vi "Expt_5_Transmitter_1.vi"() -> ()   [LabVIEW 2022 SP3]
uses:
  <instrlib>/niUSRP/niUSRP Write Tx Data (CDB).vi
  <vilib>/Analysis/NI_AALPro.lvlib
  <vilib>/measure/NI_MABase.lvlib
panel:
  out "Array 3":bool[](array[boolean])
  out "Digital Signal":dbl[](graph)
  out "Signal Without AWGN":dbl[](graph)
  out "XY Graph":cluster{i32[], i32[]}(graph)
  out "Array 2":i32[](array[numeric])
  out "Array":i32[](array[numeric])
  out "Numeric":dbl
  out "Signal With AWGN":waveform(dbl)[](graph)
  in  "active antenna":string
  in  "gain":dbl format="%#_6f"
  in  "carrier frequency":dbl=100000.0 format="%#_6p"
  in  "IQ rate":dbl=100000.0 format="%#_6p"
  in  "device names":refnum<k15>
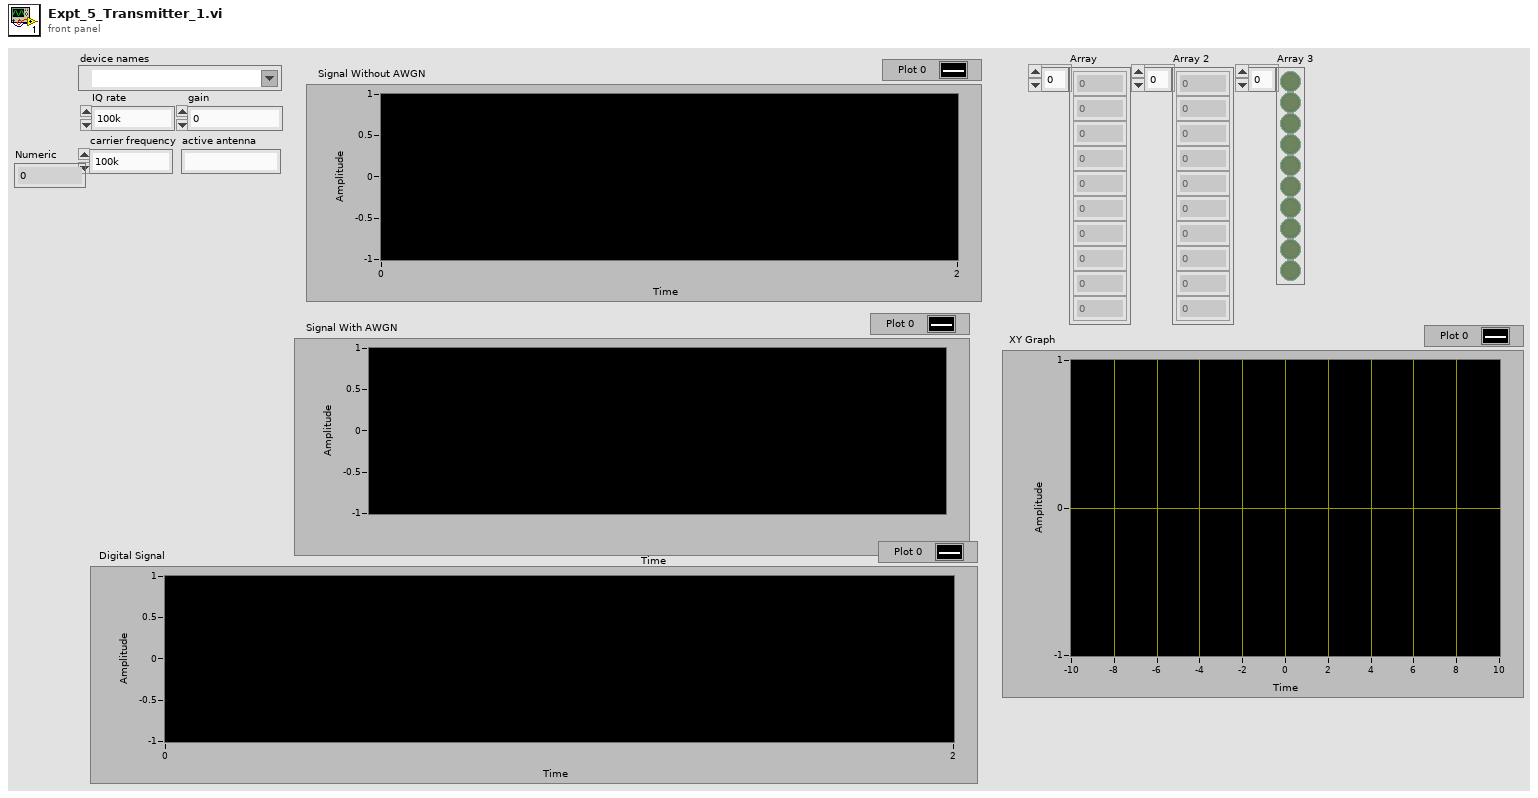
[diagram p1: front panel]
types:
  T1 = enum16{"sine", "cosine", "triangle", "square", "sawtooth", "increasing ramp", "decreasing ramp"}
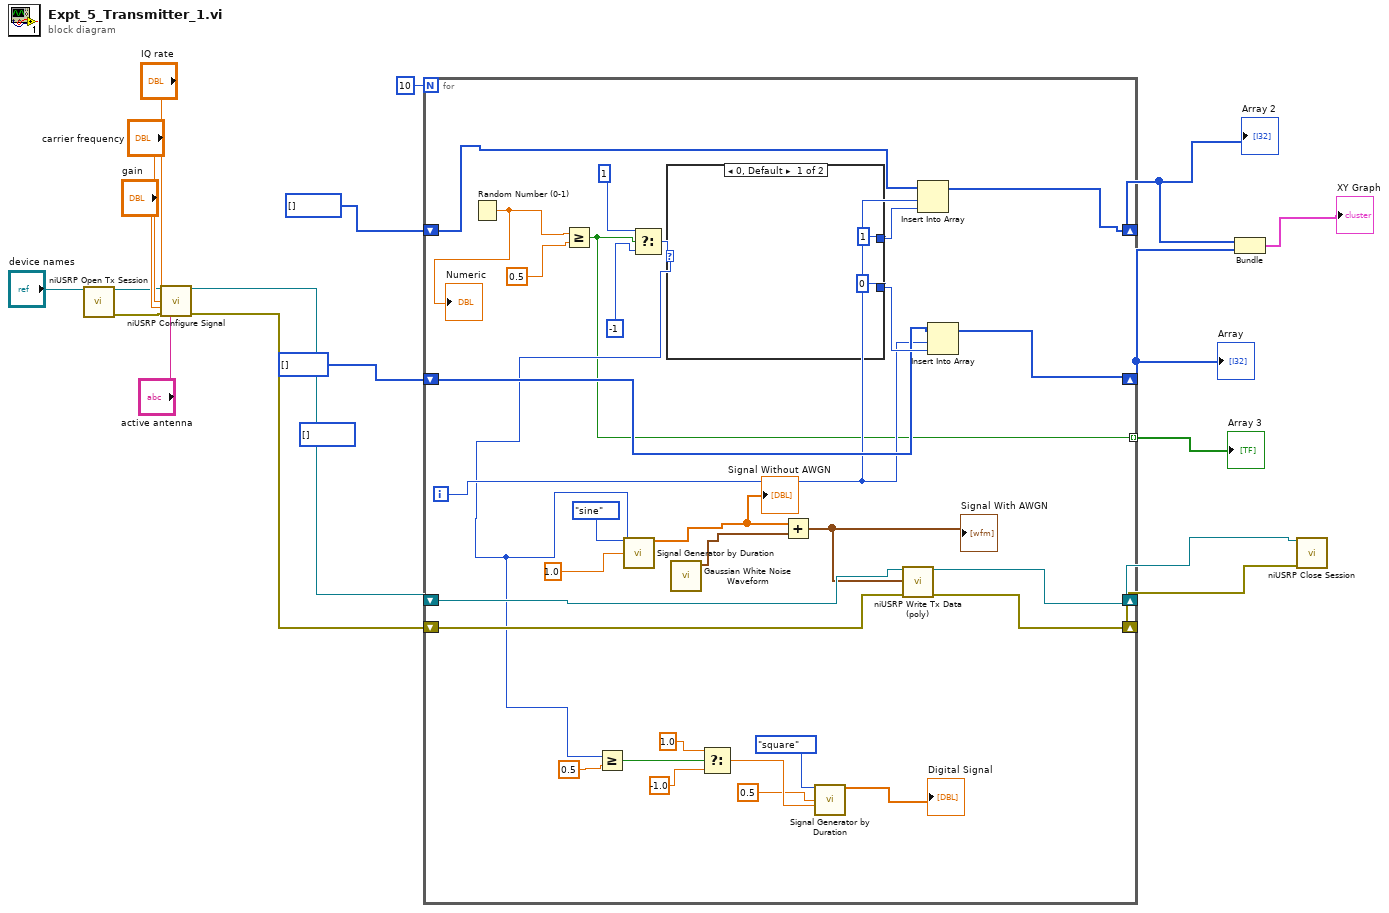
[diagram p0: block diagram]
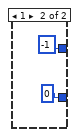
[diagram p2: hidden frame]
diagram:
  (unwired) i32[] []
  n1 = call <instrlib>:"niUSRP Open Tx Session.vi"("device names"="device names") -> ("session handle out"=w13:refnum<k15>, "error out"=w12:errorcluster)  [unwired: 13 in]
  n2 = call <instrlib>:"niUSRP Configure Signal.vi"("session handle"=w13, "IQ rate"="IQ rate", "carrier frequency"="carrier frequency", "gain"="gain", "error in (no error)"=w12, "active antenna"="active antenna") -> ("session handle out"=w6:refnum<k15>, "error out"=w5:errorcluster)  [unwired: 5 in, 3 out]
  n3 = for {
    N: 10 -> [_]
    shift-right: [w41] -> w9
    shift-left: i32[] [] -> [w43]
    shift-right: [w40] -> w8
    shift-left: i32[] [] -> [w42]
    shift-right: [w33] -> w4
    shift-left: w6 -> [w35]
    shift-right: [w32] -> w3
    shift-left: w5 -> [w34]
    tunnel: [w19] -> w2 mode=indexing
    i -> [w38]
    n4 = Random Number (0-1)() -> (number: 0 to 1=w39:dbl)
    "Numeric" <- w39
    n5 = Greater Or Equal?(x=w39, y=0.5) -> (x >= y?=w19:bool)
    n6 = Select(t=1, s=w19, f=-1) -> (s? t:f=w20:i32)
    n7 = Greater Or Equal?(x=w20, y=0.5) -> (x >= y?=w27:bool)
    n8 = call <vilib>:"Signal Generator by Duration.vi"("signal type"=T1."sine", "frequency"=1.0, "amplitude"=w20) -> ("signal"=w29:dbl[])  [unwired: 9 in, 3 out]
    "Signal Without AWGN" <- w29
    n9 = case shown="0, Default" w20 {
      tunnel: [1 -1] -> w45
      tunnel: [0 0] -> w44
      frame 0, Default {
      }
      frame 1 {
      }
    }
    n10 = call <vilib>:"Gaussian White Noise Waveform.vi"() -> ("signal out"=w31:waveform(dbl))  [unwired: 10 in, 1 out]
    n11 = Select(t=1.0, s=w27, f=-1.0) -> (s? t:f=w24:dbl)
    n12 = Add(x=w29, y=w31) -> (x+y=w30:waveform(dbl)[])
    "Signal With AWGN" <- w30
    n13 = call <vilib>:"Signal Generator by Duration.vi"("signal type"=T1."square", "frequency"=0.5, "amplitude"=w24) -> ("signal"=→"Digital Signal":dbl[])  [unwired: 9 in, 3 out]
    n14 = call-poly <instrlib>:"niUSRP Write Tx Data (poly).vi"("session handle"=w35, "data"=w30, "error in (no error)"=w34) -> ("session handle out"=w33:refnum<k15>, "error out"=w32:errorcluster)  [unwired: 11 in]
    n15 = Insert Into Array(array=w43, index=w38, new element=w45) -> (w41:i32[])
    n16 = Insert Into Array(array=w42, index=w38, new element=w44) -> (w40:i32[])
  }
  "Array" <- w8
  "Array 2" <- w9
  "Array 3" <- w2
  n17 = Bundle(w9, w8) -> (→"XY Graph":cluster{i32[], i32[]})  [unwired: 1 in]
  n18 = call <instrlib>:"niUSRP Close Session.vi"("session handle"=w4, "error in (no error)"=w3) -> ()  [unwired: 13 in, 1 out]
